vi "RT2.vi"(8 "ErrorIn":errorcluster, 10 "InCluster":T3, 11 "Reference":T1) -> (0 "ErrorOut":errorcluster, 2 "OutCluster":T2, 3 "ReferenceOut":T1)   [LabVIEW 2022 SP3]
uses:
  C:/Users/Robots/Documents/robocadSimLV/assemblies/LibraryForLabVIEW.dll
  assemblies/LibraryForLabVIEW.dll
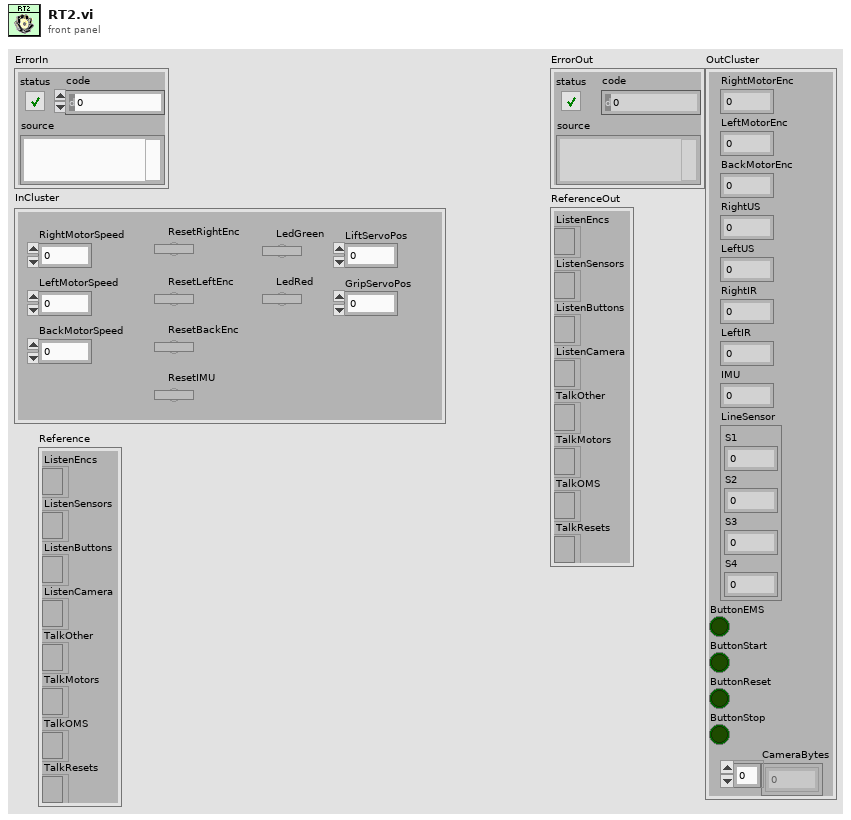
[diagram p1: front panel]
types:
  T1 = cluster{"ListenEncs":refnum<k24>, "ListenSensors":refnum<k24>, "ListenButtons":refnum<k24>, "ListenCamera":refnum<k24>, "TalkOther":refnum<k24>, "TalkMotors":refnum<k24>, "TalkOMS":refnum<k24>, "TalkResets":refnum<k24>}
  T2 = cluster{"RightMotorEnc":dbl, "LeftMotorEnc":dbl, "BackMotorEnc":dbl, "RightUS":dbl, "LeftUS":dbl, "RightIR":dbl, "LeftIR":dbl, "IMU":dbl, "LineSensor":cluster{"S1":dbl, "S2":dbl, "S3":dbl, "S4":dbl}, "ButtonEMS":bool, "ButtonStart":bool, "ButtonReset":bool, "ButtonStop":bool, "CameraBytes":u8[]}
  T3 = cluster{"RightMotorSpeed":dbl, "LeftMotorSpeed":dbl, "BackMotorSpeed":dbl, "ResetRightEnc":bool, "ResetLeftEnc":bool, "ResetBackEnc":bool, "ResetIMU":bool, "LedGreen":bool, "LedRed":bool, "LiftServoPos":dbl, "GripServoPos":dbl}
  T4 = cluster{"Encs":dbl[], "Sensors":dbl[], "Buttons":bool[], "Camera":u8[]}
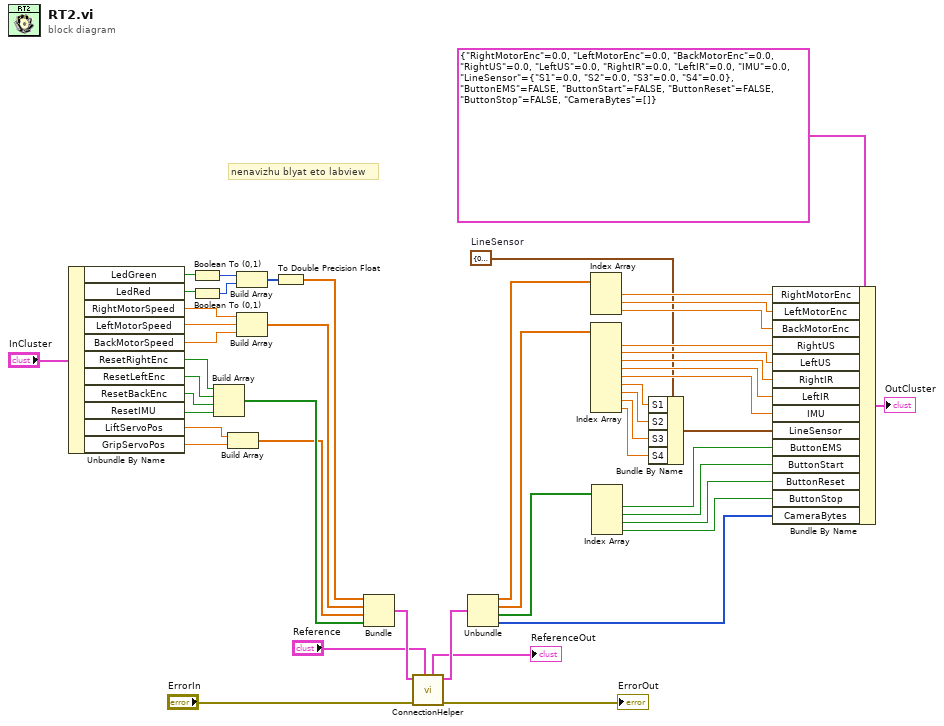
[diagram p0: block diagram]
diagram:
  w18 = cluster{"S1":dbl, "S2":dbl, "S3":dbl, "S4":dbl} {"S1"=0.0, "S2"=0.0, "S3"=0.0, "S4"=0.0}  # LineSensor
  # "nenavizhu blyat eto labview"
  n1 = Unbundle By Name("InCluster") -> ("LedGreen"=w42:bool, "LedRed"=w41:bool, "RightMotorSpeed"=w45:dbl, "LeftMotorSpeed"=w46:dbl, "BackMotorSpeed"=w44:dbl, "ResetRightEnc"=w35:bool, "ResetLeftEnc"=w36:bool, "ResetBackEnc"=w37:bool, "ResetIMU"=w38:bool, "LiftServoPos"=w3:dbl, "GripServoPos"=w2:dbl)
  n2 = Boolean To (0,1)(Boolean=w42) -> (0, 1=w40:i16)
  n3 = Boolean To (0,1)(Boolean=w41) -> (0, 1=w39:i16)
  n4 = Build Array(w35, w36, w37, w38) -> (w34:bool[])
  n5 = Build Array(w3, w2) -> (w1:dbl[])
  n6 = Build Array(w40, w39) -> (w32:i16[])
  n7 = Build Array(w45, w46, w44) -> (w43:dbl[])
  n8 = To Double Precision Float(number=w32) -> (double precision float=w31:dbl[])
  n9 = Bundle(w31, w43, w1, w34) -> (w33:cluster{dbl[], dbl[], dbl[], bool[]})  [unwired: 1 in]
  n10 = call "ConnectionHelper.vi"("Reference"="Reference", "ErrorIn"="ErrorIn", "InCluster"=w33) -> ("ErrorOut"=→"ErrorOut":errorcluster, "OutCluster"=w30:T4, "ReferenceOut"=→"ReferenceOut":T1)  [unwired: 6 in]
  n11 = Unbundle(w30) -> ("Encs"=w29:dbl[], "Sensors"=w24:dbl[], "Buttons"=w12:bool[], "Camera"=w8:u8[])
  n12 = Index Array(array=w29) -> (element #1=w27:dbl, element #2=w26:dbl, element #3=w25:dbl)  [unwired: 3 in]
  n13 = Index Array(array=w24) -> (element #1=w23:dbl, element #2=w22:dbl, element #3=w21:dbl, element #4=w20:dbl, element #5=w19:dbl, element #6=w16:dbl, element #7=w15:dbl, element #8=w14:dbl, element #9=w13:dbl)  [unwired: 9 in]
  n14 = Index Array(array=w12) -> (element #1=w11:bool, element #2=w10:bool, element #3=w9:bool, element #4=w6:bool)  [unwired: 4 in]
  n15 = Bundle By Name(cluster=w18, "S1"=w16, "S2"=w15, "S3"=w14, "S4"=w13) -> (w17:cluster{"S1":dbl, "S2":dbl, "S3":dbl, "S4":dbl})
  n16 = Bundle By Name(cluster=T2 {"RightMotorEnc"=0.0, "LeftMotorEnc"=0.0, "BackMotorEnc"=0.0, "RightUS"=0.0, "LeftUS"=0.0, "RightIR"=0.0, "LeftIR"=0.0, "IMU"=0.0, "LineSensor"={"S1"=0.0, "S2"=0.0, "S3"=0.0, "S4"=0.0}, "ButtonEMS"=FALSE, "ButtonStart"=FALSE, "ButtonReset"=FALSE, "ButtonStop"=FALSE, "CameraBytes"=[]} ("input cluster"), "RightMotorEnc"=w27, "LeftMotorEnc"=w26, "BackMotorEnc"=w25, "RightUS"=w23, "LeftUS"=w22, "RightIR"=w21, "LeftIR"=w20, "IMU"=w19, "LineSensor"=w17, "ButtonEMS"=w11, "ButtonStart"=w10, "ButtonReset"=w9, "ButtonStop"=w6, "CameraBytes"=w8) -> (→"OutCluster":T2)
